vi "10 AttributeGet.vi"(8 "error in (no error)":errorcluster caption="错误输入（无错误）", 11 "SerialClass 输入":refnum<class "SerialClass.lvclass">) -> (0 "error out":errorcluster caption="错误输出", 1 "串口名称":string, 2 "串口配置":T1={"VISA串口名称"="", "波特率"=9600, "停止位"=10, "流控制"=0, "数据位"=8, "奇偶校验"=enum."None", "超时"=2000, "启用终止符？"=FALSE, "终止符"=10} {"终止符" format="%.0x"; "数据位" min=5 max=8 step=1; "流控制" items=["无", "XON/XOFF", "RTS/CTS", "XON/XOFF & RTS/CTS", "DTR/DSR", "XON/XOFF & DTR/DSR"]; "停止位" items=["1.0"=10, "1.5"=15, "2.0"=20]; "波特率" items=["9600"=9600, "115200"=15]}, 3 "SerialClass 输出":refnum<class "SerialClass.lvclass">)   [LabVIEW 2019, in "SerialClass.lvclass"]
uses:
  SerialClass.lvclass
  00 Ctl/SerialData.ctl
  SerialClass.lvclass/SerialClass.ctl
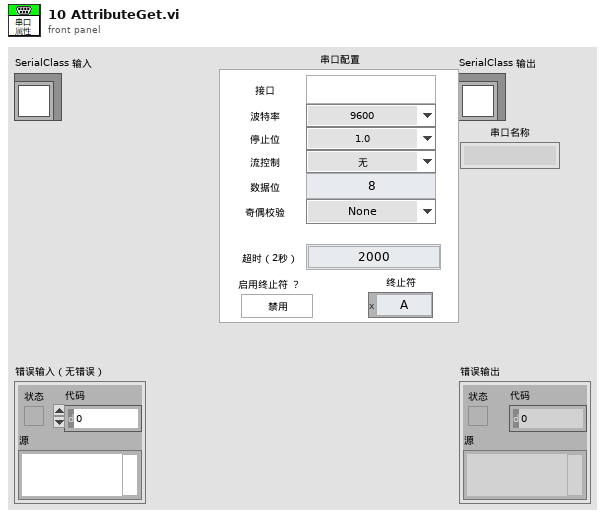
[diagram p1: front panel]
types:
  T1 = typedef "SerialData.ctl" = cluster{"VISA串口名称":refnum<visa-resource-name>, "波特率":u32, "停止位":u16, "流控制":u16, "数据位":u16, "奇偶校验":enum16{"None", "Odd", "Even", "Mark", "Space"}, "超时":u32, "启用终止符？":bool, "终止符":u8}
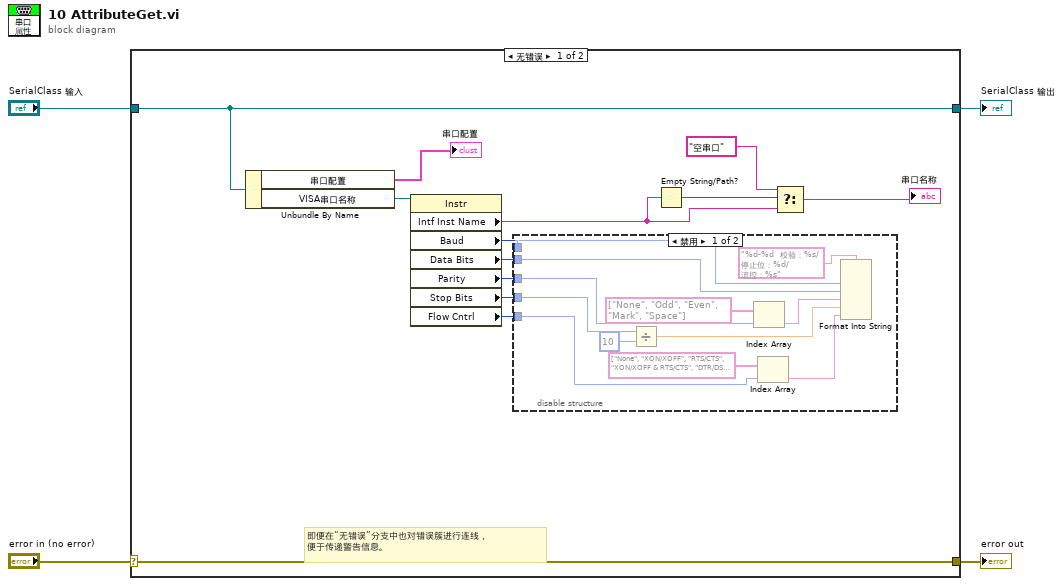
[diagram p0: block diagram]
diagram:
  n1 = case shown="无错误" "error in (no error)" {
    selector: "error in (no error)" -> [w17 w31]
    tunnel: [w17 w31] -> w3
    tunnel: [w16 w30] -> w1
    tunnel: "SerialClass 输入" -> [w16 w30]
    frame No Error {
      # "即便在“无错误”分支中也对错误簇进行连线，\n便于传递警告信息。"
      n2 = Unbundle By Name(w16) -> ("串口配置"=→"串口配置":T1, "VISA串口名称"=w5:refnum<visa-resource-name>)
      n3 = property class="Instr"(reference=w5) -> ("Intf Inst Name"=w15:string, "Baud"=w9:u32, "Data Bits"=w10:u16, "Parity"=w11:u16, "Stop Bits"=w13:u16, "Flow Cntrl"=w12:u16)  [unwired: 1 in, 2 out]
      n4 = disable-structure shown="禁用" {
        disable-tunnel: w13 -> [w28 _]
        disable-tunnel: w12 -> [w26 _]
        disable-tunnel: w11 -> [w25 _]
        disable-tunnel: w10 -> [w23 _]
        disable-tunnel: w9 -> [w22 _]
        frame Disabled {
          n5 = Divide(x=w28, y=u16 10) -> (x/y=w29:dbl)
          n6 = Index Array(array=string[] ["None", "Odd", "Even", "Mark", "Space"] ("校验"), index=w25) -> (element=w24:string)
          n7 = Index Array(array=string[] ["None", "XON/XOFF", "RTS/CTS", "XON/XOFF & RTS/CTS", "DTR/DSR", "XON/XOFF & DTR/DSR"] ("流控"), index=w26) -> (element=w27:string)
          n8 = Format Into String(format string="%d-%d  校验：%s/停止位：%d/流控：%s" ("格式字符串"), w22, w23, w24, w29, w27) -> ()  [unwired: 2 in, 2 out]
        }
        frame Enabled {
        }
      }
      n9 = Empty String/Path?(string/path=w15) -> (empty?=w14:bool)
      n10 = Select(t="空串口", s=w14, f=w15) -> (s? t:f=→"串口名称":string)
    }
    frame Error {
    }
  }
  "error out" <- w3
  "SerialClass 输出" <- w1
